vi "边沿产生.vi"(3 "RST":bool, 4 "IN":bool, 5 "EN":bool=TRUE) -> (0 "PLF":bool, 1 "Edge":bool, 2 "PLS":bool)   [LabVIEW 2018]
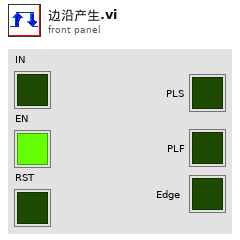
[diagram p1: front panel]
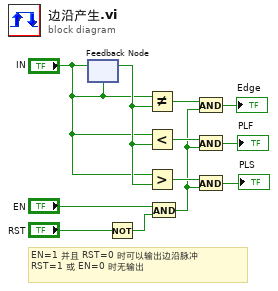
[diagram p0: block diagram]
diagram:
  # "EN=1 并且 RST=0 时可以输出边沿脉冲\nRST=1 或 EN=0 时无输出"
  n1 = feedback-in #1("IN") -> ()
  n2 = feedback #1("IN") -> (w12:bool)
  n3 = Not(x="RST") -> (.not. x?=w2:bool)
  n4 = Not Equal?(x="IN", y=w12) -> (x != y?=w10:bool)
  n5 = Less?(x="IN", y=w12) -> (x < y?=w9:bool)
  n6 = Greater?(x="IN", y=w12) -> (0:w8:bool)
  n7 = And(x="EN", y=w2) -> (x .and. y?=w3:bool)
  n8 = And(x=w10, y=w3) -> (x .and. y?=→"Edge":bool)
  n9 = And(x=w9, y=w3) -> (x .and. y?=→"PLF":bool)
  n10 = And(x=w8, y=w3) -> (x .and. y?=→"PLS":bool)
